vi "SPD.HV_bias Range.vi"(5 "Continue":refnum<vi>, 7 "Progress":refnum<vi>, 8 "Error In":errorcluster, 10 "HV_GridParams":T1, 11 "SPD.Stand Ctrl in":T2 {"spdDeviceSession"."hidSPD.Controller"."HV_bias" format="%#_6p, V"; "spdDeviceSession"."hidSPD.Controller"."TSet" format="%#_6p, DegC"}) -> (0 "Error Out":errorcluster, 1 "done":bool, 3 "SPD.Stand Ctrl out":T2 {"spdDeviceSession"."hidSPD.Controller"."HV_bias" format="%#_6p, V"; "spdDeviceSession"."hidSPD.Controller"."TSet" format="%#_6p, DegC"})   [LabVIEW 2018]
uses:
  typedefs/SPD.Stand Ctrl.ctl
  Instruments/SPD HID Interface/hidSPDLibForLabView/LibVIs/hidSPD Controls/hidSPD Device Session.ctl
  Instruments/SPD HID Interface/hidSPDLibForLabView/LibVIs/hidSPD Controls/hidSPD Controller.ctl
  Instruments/KC705 DevBoard/typedefs/DevB.Session.ctl
  Instruments/KeySight 53230A/typedefs/FreqC.Session.ctl
  Instruments/KeySight 8164B/KeySight 8164B LAN InstrLib/typedefs/KeySight 8164B control.ctl
  Instruments/LeCroy SDA830/typedefs/LeCroy.Session.ctl
  typedefs/SPD.Events.ctl
  <vilib>/Utility/config.llb/Config Data RefNum.ctl
  typedefs/SPD.Meas Result.ctl
  SPD.HV_Grid Test Params.ctl
  HV_Grid Range Search States.ctl
  SubVIs/Min_Max.ctl
  SubVIs/comparison mode.ctl
  <vilib>/Analysis/1siggen.llb/Ramp Pattern by Samples.vi
  Instruments/KeySight 8164B/KeySight 8164B LAN InstrLib.lvlib
  <vilib>/Analysis/NI_AALBase.lvlib
  Instruments/SPD HID Interface/hidSPDLibForLabView/hidSPDLibForLabView.lvlib
  <vilib>/Utility/config.llb/NI_LVConfig.lvlib
panel:
  out "Numeric 2":i32
  out "Numeric":i32
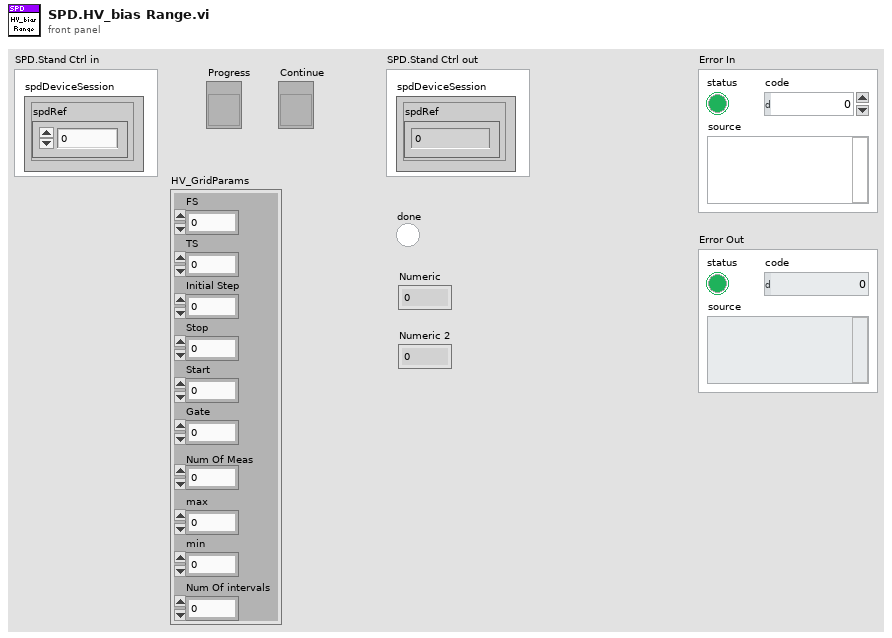
[diagram p1: front panel]
types:
  T1 = typedef "SPD.HV_Grid Test Params.ctl" = cluster{"FS":i32, "TS":i32, "Initial Step":dbl, "Stop":dbl, "Start":dbl, "Gate":dbl, "Num Of Meas":i32, "max":dbl, "min":dbl, "Num Of intervals":i32}
  T2 = typedef "SPD.Stand Ctrl.ctl" = cluster{"spdDeviceSession":T3, "DevBSession":T5, "FreqCSession":T6, "8164BSession":T7, "LeCroySession":T8, "Events":T9, "configFile":T10, "SPD.Result":T11}
  T3 = typedef "hidSPDLibForLabView.lvlib/hidSPD Device Session.ctl" = cluster{"spdRef":u64, "connected":bool, "spdName":string, "hidSPD.Controller":T4}
  T4 = typedef "hidSPDLibForLabView.lvlib/hidSPD Controller.ctl" = cluster{"TSet":sgl, "HV_bias":sgl, "DDS_stb_code":u16}
  T5 = typedef "DevB.Session.ctl" = cluster{"DevBRef":refnum<visa-resource-name>, "connected":bool}
  T6 = typedef "FreqC.Session.ctl" = cluster{"FreqCRef":refnum<visa-resource-name>, "timeout":dbl, "Gate":dbl, "connected":bool}
  T7 = typedef "KeySight 8164B LAN InstrLib.lvlib/KeySight 8164B control.ctl" = cluster{"Connection ID":refnum<k5>, "Connected":bool, "Info":string, "Slots Info":string[]}
  T8 = typedef "LeCroy.Session.ctl" = cluster{"LeCroySession":refnum<visa-resource-name>, "connected":bool}
  T9 = typedef "SPD.Events.ctl" = cluster{"DCRTest":refnum<user-event>, "Stop":refnum<user-event>}
  T10 = typedef "NI_LVConfig.lvlib/Config Data RefNum.ctl" = refnum<k1>
  T11 = typedef "SPD.Meas Result.ctl" = cluster{"HV_Bias":dbl[][][], "Stb_code":dbl[], "Temprature":dbl[], "Data":dbl[][][][]}
  T12 = typedef "Min_Max.ctl" = cluster{"min":dbl, "max":dbl}
  T13 = typedef "HV_Grid Range Search States.ctl" = enum16{"in range", "max", "min"}
  T14 = typedef "comparison mode.ctl" = enum16{"in range", "bigger then min", "bigger then max", "less then min", "less then max"}
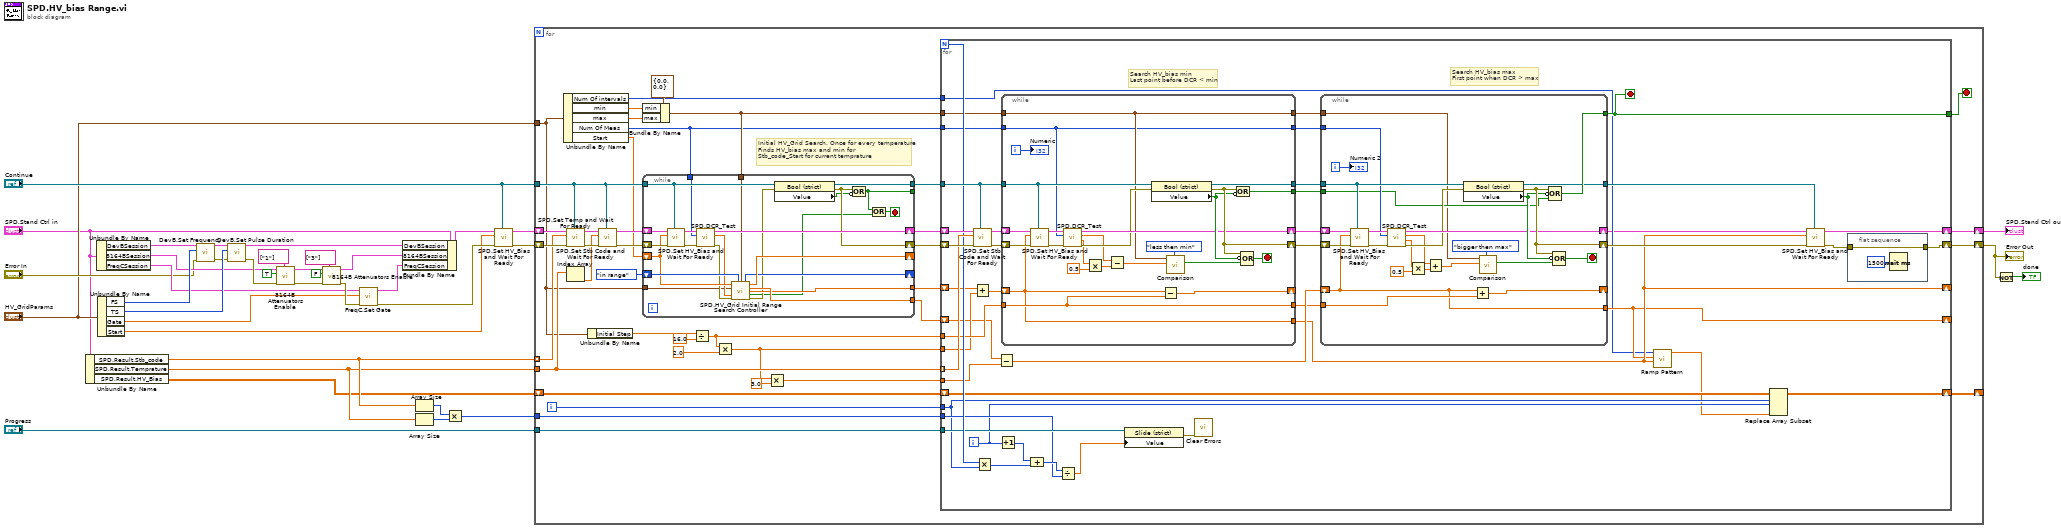
[diagram p0: block diagram]
diagram:
  n1 = Unbundle By Name("SPD.Stand Ctrl in") -> ("SPD.Result.Stb_code"=w3:dbl[], "SPD.Result.Temprature"=w2:dbl[], "SPD.Result.HV_Bias"=w1:dbl[][][])
  n2 = Unbundle By Name("SPD.Stand Ctrl in") -> ("DevBSession"=w38:T5, "8164BSession"=w25:T7, "FreqCSession"=w24:T6)
  n3 = Unbundle By Name("HV_GridParams") -> ("FS"=w36:i32, "TS"=w35:i32, "Gate"=w13:dbl, "Start"=w8:dbl)
  n4 = call "DevB.Set Frequency.vi"("error in (no error)"="Error In", "Frequency"=w36, "DevB Session in"=w38) -> ("error out"=w34:errorcluster, "DevB Session out"=w37:T5)  [unwired: 7 in]
  n5 = call "DevB.Set Pulse Duration.vi"("error in (no error)"=w34, "Pulse Duration"=w35, "DevB Session in"=w37) -> ("error out"=w27:errorcluster, "DevB Session out"=w23:T5)  [unwired: 7 in]
  n6 = call "8164B Attenuators Enable.vi"("Slots"=string[] ["1"], "error in"=w27, "Enable"=TRUE, "KeySight 8164B control in"=w25) -> ("error out"=w31:errorcluster, "KeySight 8164B control out"=w30:T7)  [unwired: 6 in]
  n7 = call "8164B Attenuators Enable.vi"("Slots"=string[] ["3"], "error in"=w31, "Enable"=FALSE, "KeySight 8164B control in"=w30) -> ("error out"=w26:errorcluster, "KeySight 8164B control out"=w22:T7)  [unwired: 6 in]
  n8 = call "FreqC.Set Gate.vi"("error In"=w26, "Gate, sec"=w13, "FreqC Session in"=w24) -> ("error out"=w12:errorcluster, "FreqC Session out"=w21:T6)  [unwired: 7 in]
  n9 = Bundle By Name(cluster="SPD.Stand Ctrl in", "DevBSession"=w23, "8164BSession"=w22, "FreqCSession"=w21) -> (w5:T2)
  n10 = Array Size(array=w3) -> (size(s)=w20:i32)
  n11 = Array Size(array=w2) -> (size(s)=w19:i32)
  n12 = Multiply(x=w20, y=w19) -> (x*y=w18:i32)
  n13 = call "SPD.Set HV_Bias and Wait For Ready.vi"("Continue"="Continue", "Error In"=w12, "HV_Bias"=w8, "SPD.Stand Ctrl in"=w5) -> ("Error Out"=w10:errorcluster, "SPD.Stand Ctrl out"=w11:T2)  [unwired: 6 in]
  n14 = for {
    shift-right: [w77] -> w17
    shift-left: w11 -> [w75]
    tunnel: w2 -> [w66]
    tunnel: w3 -> [w73] mode=indexing
    shift-right: [w76] -> w15
    shift-left: w10 -> [w74]
    tunnel: "Continue" -> [w62]
    tunnel: w18 -> [w70]
    tunnel: "Progress" -> [w69]
    tunnel: "HV_GridParams" -> [w47]
    shift-right: [w39] -> _
    shift-left: w1 -> [w40]
    i -> [w71]
    stop <- w72 stop-if-true
    # "Initial HV_Grid Search. Once for every temperature\nFinds HV_bias max and min for \nStb_code_Start for current temprature"
    n15 = Unbundle By Name(w47) -> ("Num Of intervals"=w44:i32, "min"=w50:dbl, "max"=w49:dbl, "Num Of Meas"=w48:i32, "Start"=w53:dbl)
    n16 = call "SPD.Set Temp and Wait For Ready.vi"("Continue"=w62, "Error In"=w74, "Tset"=w73, "SPD.Stand Ctrl in"=w75) -> ("Error Out"=w67:errorcluster, "SPD.Stand Ctrl out"=w68:T2)  [unwired: 6 in]
    n17 = Index Array(array=w66) -> (element=w65:dbl)  [unwired: 1 in]
    n18 = Unbundle By Name(w47) -> ("Initial Step"=w46:dbl)
    n19 = call "SPD.Set Stb Code and Wait For Ready.vi"("Continue"=w62, "Error In"=w67, "Strobe code"=w65, "SPD.Stand Ctrl in"=w68) -> ("Error Out"=w63:errorcluster, "SPD.Stand Ctrl out"=w64:T2)  [unwired: 6 in]
    n20 = Bundle By Name(cluster=T12 {"min"=0.0, "max"=0.0} ("minMax"), "min"=w50, "max"=w49) -> (w51:T12)
    n21 = while {
      tunnel: w62 -> [w88]
      shift-right: [w85] -> w57
      shift-left: w63 -> [w100]
      shift-right: [w97] -> _
      shift-left: w53 -> [w94]
      shift-right: [w95] -> _
      shift-left: HV_Grid_Range_Search_States."in range" ("next state") -> [w96]
      shift-right: [w91] -> w58
      shift-left: w64 -> [w101]
      tunnel: [w90] -> w56
      tunnel: [w89] -> w55
      tunnel: [w86] -> w59
      tunnel: [w82] -> _
      tunnel: w51 -> [w80]
      tunnel: w48 -> [w79]
      tunnel: w47 -> [w78]
      stop <- w83 stop-if-true
      n22 = call "SPD.Set HV_Bias and Wait For Ready.vi"("Continue"=w88, "Error In"=w100, "HV_Bias"=w94, "SPD.Stand Ctrl in"=w101) -> ("Error Out"=w99:errorcluster, "SPD.Stand Ctrl out"=w98:T2)  [unwired: 6 in]
      n23 = call "SPD.DCR_Test.vi"("Error In"=w99, "Num of Meas"=w79, "SPD.Stand Ctrl in"=w98) -> ("Error Out"=w92:errorcluster, "DCR"=w93:dbl, "SPD.Stand Ctrl out"=w91:T2)  [unwired: 5 in, 1 out]
      n24 = call "SPD.HV_Grid Initial Range Search Controller.vi"("HV_bias"=w94, "state"=w96, "DCRRange"=w80, "HV_GridParams"=w78, "DCR"=w93, "Error In"=w92) -> ("next state"=w95:T13, "HV_bias Next"=w97:dbl, "HV_bias max"=w90:dbl, "HV_bias min"=w89:dbl, "done"=w81:bool, "Error Out"=w87:errorcluster)  [unwired: 4 in]
      n25 = property class="Bool (strict)"(reference=w88, error in=w87) -> (reference out=w86:refnum<vi>, error out=w85:errorcluster, "Value"=w84:bool)
      n26 = Compound Arithmetic op=OR(w85, invert w84) -> (w82:bool)
      n27 = Compound Arithmetic op=OR(w82, w81) -> (w83:bool)
    }
    n28 = Divide(x=w46, y=16.0) -> (x/y=w54:dbl)
    n29 = Multiply(x=w54, y=2.0) -> (x*y=w43:dbl)
    n30 = Multiply(x=w43, y=3.0) -> (x*y=w41:dbl)
    n31 = for {
      N -> [w140]
      tunnel: w66 -> [w142] mode=indexing
      shift-right: [w118] -> w77
      shift-left: w58 -> [w146]
      shift-right: [w109] -> w76
      shift-left: w57 -> [w144]
      tunnel: w59 -> [w141]
      tunnel: [w123] -> w72
      tunnel: w71 -> [w104]
      tunnel: w70 -> [w133]
      tunnel: w69 -> [w134]
      tunnel: w48 -> [w127]
      shift-right: [w112] -> _
      shift-left: w56 -> [w114]
      shift-right: [w113] -> _
      shift-left: w55 -> [w115]
      tunnel: w54 -> [w125]
      tunnel: w51 -> [w131]
      tunnel: w43 -> [w121]
      tunnel: w44 -> [w111]
      tunnel: w41 -> [w108]
      shift-right: [w105] -> w39
      shift-left: w40 -> [w107]
      i -> [w103]
      stop <- w123 stop-if-true
      # "Search HV_bias max\nFirst point when DCR > max"
      # "Search HV_bias min\nLast point before DCR < min"
      n32 = call "SPD.Set Stb Code and Wait For Ready.vi"("Continue"=w141, "Error In"=w144, "Strobe code"=w142, "SPD.Stand Ctrl in"=w146) -> ("Error Out"=w143:errorcluster, "SPD.Stand Ctrl out"=w145:T2)  [unwired: 6 in]
      n33 = Add(x=w115, y=w121) -> (x+y=w132:dbl)
      n34 = Multiply(x=w140, y=w104) -> (x*y=w135:i32)
      n35 = Subtract(x=w114, y=w108) -> (x-y=w126:dbl)
      n36 = Increment(x=w103) -> (x+1=w136:i32)
      n37 = while {
        shift-right: [w165] -> w128
        shift-left: w145 -> [w173]
        shift-right: [w168] -> w119
        shift-left: w143 -> [w171]
        tunnel: w141 -> [w170]
        tunnel: [w169] -> w124
        tunnel: w127 -> [w157]
        shift-right: [w163] -> _
        shift-left: w132 -> [w154]
        tunnel: w131 -> [w159]
        tunnel: w125 -> [w156]
        tunnel: [w154] -> w113
        tunnel: [w159] -> w130
        tunnel: [w158] -> w129
        tunnel: [w157] -> w122
        tunnel: [w156] -> w120
        i -> [w155]
        stop <- w166 stop-if-true
        n38 = call "SPD.Set HV_Bias and Wait For Ready.vi"("Continue"=w170, "Error In"=w171, "HV_Bias"=w154, "SPD.Stand Ctrl in"=w173) -> ("Error Out"=w164:errorcluster, "SPD.Stand Ctrl out"=w172:T2)  [unwired: 6 in]
        n39 = call "SPD.DCR_Test.vi"("Error In"=w164, "Num of Meas"=w157, "SPD.Stand Ctrl in"=w172) -> ("Error Out"=w160:errorcluster, "DCR sigma"=w150:dbl, "DCR"=w153:dbl, "SPD.Stand Ctrl out"=w165:T2)  [unwired: 5 in]
        n40 = Multiply(x=w150, y=0.5) -> (x*y=w151:dbl)
        n41 = Subtract(x=w153, y=w151) -> (x-y=w152:dbl)
        n42 = property class="Bool (strict)"(reference=w170, error in=w160) -> (reference out=w158:refnum<vi>, error out=w168:errorcluster, "Value"=w167:bool)
        n43 = Subtract(x=w154, y=w156) -> (x-y=w163:dbl)
        n44 = call "Comparison.vi"("Comparison Mode"=comparison_mode."less then min", "value"=w152, "minMax"=w159) -> ("result"=w161:bool)  [unwired: 8 in]
        n45 = Compound Arithmetic op=OR(w168, invert w167) -> (w169:bool)
        n46 = Compound Arithmetic op=OR(w168, invert w167, w161) -> (w166:bool)
        "Numeric" <- w155
      }
      n47 = Compound Arithmetic op=ADD(w136, w135) -> (w137:i32)
      n48 = Divide(x=w137, y=w133) -> (x/y=w138:dbl)
      n49 = property class="Slide (strict)"(reference=w134, "Value"=w138) -> (error out=w139:errorcluster)  [unwired: 1 in, 1 out]
      n50 = call <vilib>:"Clear Errors.vi"("error in (no error)"=w139) -> ()  [unwired: 5 in, 2 out]
      n51 = while {
        shift-right: [w191] -> w106
        shift-left: w128 -> [w199]
        shift-right: [w194] -> w116
        shift-left: w119 -> [w197]
        tunnel: w129 -> [w196]
        tunnel: [w195] -> w123
        tunnel: w122 -> [w189]
        shift-right: [w187] -> _
        shift-left: w126 -> [w183]
        tunnel: w130 -> [w180]
        tunnel: w120 -> [w188]
        tunnel: [w183] -> w112
        tunnel: w124 -> [w182]
        tunnel: [w181] -> w117
        i -> [w179]
        stop <- w192 stop-if-true
        n52 = call "SPD.Set HV_Bias and Wait For Ready.vi"("Continue"=w196, "Error In"=w197, "HV_Bias"=w183, "SPD.Stand Ctrl in"=w199) -> ("Error Out"=w190:errorcluster, "SPD.Stand Ctrl out"=w198:T2)  [unwired: 6 in]
        n53 = call "SPD.DCR_Test.vi"("Error In"=w190, "Num of Meas"=w189, "SPD.Stand Ctrl in"=w198) -> ("Error Out"=w184:errorcluster, "DCR sigma"=w174:dbl, "DCR"=w175:dbl, "SPD.Stand Ctrl out"=w191:T2)  [unwired: 5 in]
        n54 = Multiply(x=w174, y=0.5) -> (x*y=w178:dbl)
        n55 = Add(x=w175, y=w178) -> (x+y=w176:dbl)
        n56 = property class="Bool (strict)"(reference=w196, error in=w184) -> (reference out=w181:refnum<vi>, error out=w194:errorcluster, "Value"=w193:bool)
        n57 = Add(x=w183, y=w188) -> (x+y=w187:dbl)
        n58 = call "Comparison.vi"("Comparison Mode"=comparison_mode."bigger then max", "value"=w176, "minMax"=w180) -> ("result"=w185:bool)  [unwired: 8 in]
        n59 = Compound Arithmetic op=OR(w194, invert w193, w182) -> (w195:bool)
        n60 = Compound Arithmetic op=OR(w194, invert w193, w185) -> (w192:bool)
        "Numeric 2" <- w179
      }
      n61 = call-poly <vilib>:"Ramp Pattern.vi"("start"=w113, "end"=w112, "samples"=w111) -> ("Ramp Pattern"=w102:dbl[])  [unwired: 7 in, 1 out]
      n62 = Replace Array Subset(array=w107, new element=w102, index (dim 0)=w104, index (dim 1)=w103) -> (w105:dbl[][][])  [unwired: 1 in]
      n63 = call "SPD.Set HV_Bias and Wait For Ready.vi"("Continue"=w117, "Error In"=w116, "HV_Bias"=w113, "SPD.Stand Ctrl in"=w106) -> ("Error Out"=w110:errorcluster, "SPD.Stand Ctrl out"=w118:T2)  [unwired: 6 in]
      n64 = flat-sequence {
        tunnel: w110 -> [w148]
        tunnel: [w148] -> w109
        frame #0 {
          n65 = Wait (ms)(milliseconds to wait=u32 1500) -> ()  [unwired: 1 out]
        }
      }
    }
  }
  "SPD.Stand Ctrl out" <- w17
  "Error Out" <- w15
  n66 = Not(x=w15) -> (.not. x?=→"done":bool)
